vi "Get Operation System Version(冲突时的文件备份2013-03-27 14-07-26).vi"(8 "错误输入（无错误）":errorcluster) -> (0 "错误输出":errorcluster, 3 "Operation System":T1)   [LabVIEW 2012, in "Application.lvlib"]
uses:
  Application.lvlib
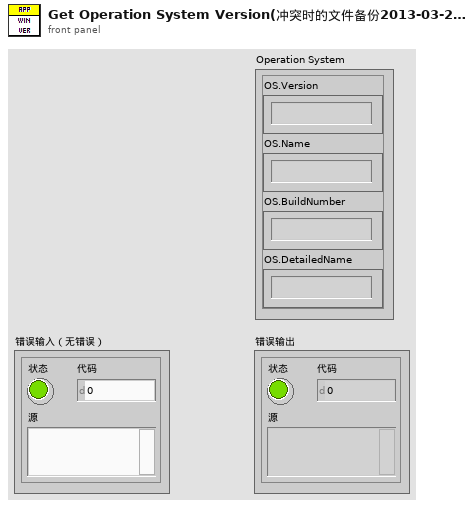
[diagram p1: front panel]
types:
  T1 = cluster{"OS.Version":string, "OS.Name":string, "OS.BuildNumber":string, "OS.DetailedName":string}
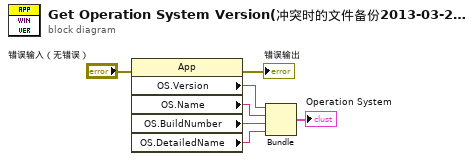
[diagram p0: block diagram]
diagram:
  n1 = property class="App"(error in="错误输入（无错误）") -> (error out=→"错误输出":errorcluster, "OS.Version"=w7:string, "OS.Name"=w6:string, "OS.BuildNumber"=w5:string, "OS.DetailedName"=w4:string)  [unwired: 1 in, 1 out]
  n2 = Bundle("OS.Version"=w7, "OS.Name"=w6, "OS.BuildNumber"=w5, "OS.DetailedName"=w4) -> (→"Operation System":T1)  [unwired: 1 in]
